vi "onStop.vi"(8 "error in (no error)":errorcluster, 11 "MAUI":refnum<class "MAUI.lvclass">) -> (0 "error out":errorcluster, 3 "MAUI out":refnum<class "MAUI.lvclass">)   [LabVIEW 2019, in "MAUI.lvclass"]
doc: "JKI State Machine Objects (SMO) 1.3.0.56\nJKI - JKI\nCopyright (c) 2017, JKI"
uses:
  MAUI.lvclass
  <userlib>/LevyLab/Embedded UI/SMO.UI.Embedded/Embedded UI.lvclass
  C:/Program Files (x86)/National Instruments/LabVIEW 2019/vi.lib/JKI/JKI SMO/SMO/SMO.lvclass
  <vilib>/JKI/JKI SMO/SMO.UI/SMO.UI.lvclass
  <vilib>/JKI/JKI SMO/SMO/SMO.lvclass
panel:
  # "For instructions on how to use the JKI State Machine Objects, examples and video tutorials, visit:\nhttp://jki.net/state-machine-objects/\n\nJKI State Machine Objects™\nhttp://jki.net/state-machine-objects/\nCopyright (C) 2005-2015, JKI <info@jki.net>\nALL RIGHTS RESERVED"
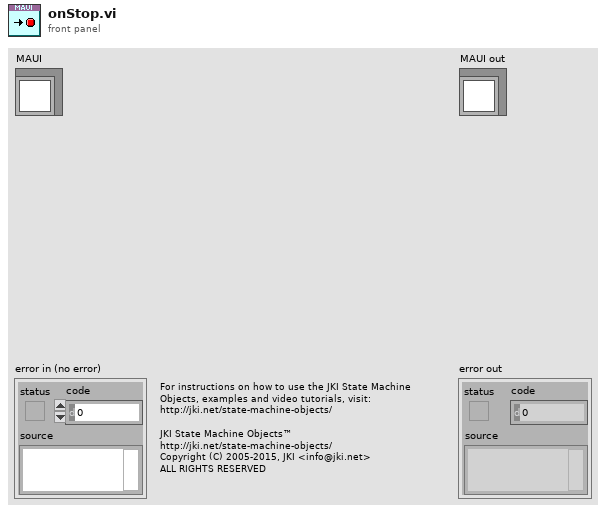
[diagram p1: front panel]
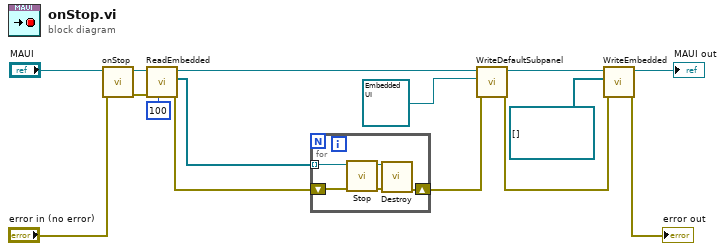
[diagram p0: block diagram]
diagram:
  n1 = call-parent "onStop.vi"("error in (no error)"="error in (no error)", "SMO"="MAUI") -> ("error out"=w14:errorcluster, "SMO out"=w9:refnum<class "MAUI.lvclass">)  [unwired: 8 in]
  n2 = call "ReadEmbedded.vi"("timeout in ms (-1)"=100, "error in (no error)"=w14, "MAUI in"=w9) -> ("error out"=w1:errorcluster, "Subpanels"=w2:refnum<class "Embedded UI.lvclass">[], "MAUI out"=w3:refnum<class "MAUI.lvclass">)  [unwired: 6 in]
  n3 = for {
    shift-right: [w18] -> w12
    shift-left: w1 -> [w20]
    tunnel: w2 -> [w17] mode=indexing
    n4 = call <vilib>:"Stop.vi"("error in (no error)"=w20, "SMO"=w17) -> ("error out"=w19:errorcluster, "SMO out"=w16:refnum<class "Embedded UI.lvclass">)  [unwired: 8 in]
    n5 = call <vilib>:"Destroy.vi"("error in (no error)"=w19, "SMO"=w16) -> ("error out"=w18:errorcluster)  [unwired: 9 in]
  }
  n6 = call "WriteDefaultSubpanel.vi"("error in (no error)"=w12, "SMO.UI.Embedded"=refnum<class "Embedded UI.lvclass"> refnum, "SMO.UI.MAUI in"=w3) -> ("error out"=w11:errorcluster, "SMO.UI.MAUI out"=w4:refnum<class "MAUI.lvclass">)  [unwired: 7 in]
  n7 = call "WriteEmbedded.vi"("error in (no error)"=w11, "Subpanels"=refnum<class "Embedded UI.lvclass">[] [], "MAUI in"=w4) -> ("error out"=→"error out":errorcluster, "MAUI out"=→"MAUI out":refnum<class "MAUI.lvclass">)  [unwired: 7 in]
